vi "Multify(DBL[]).vi"(1 "启用（T）":bool=TRUE, 2 "In":dbl[](array[numeric]), 4 "n":dbl=1.0) -> (6 "Out":dbl[](array[numeric]) format="%.2f")   [LabVIEW 2011]
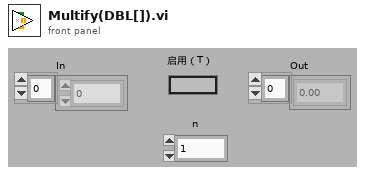
[diagram p1: front panel]
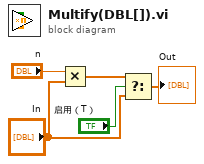
[diagram p0: block diagram]
diagram:
  n1 = Multiply(x="n", y="In") -> (x*y=w1:dbl[])
  n2 = Select(t=w1, s="启用（T）", f="In") -> (s? t:f=→"Out":dbl[])
